vi "Measurement Logic.vi"() -> ()   [LabVIEW 2021, in "audio_frequencyResponseMeasurement.lvlib"]
uses:
  audio_frequencyResponseMeasurement.lvlib
  <vilib>/addons/_NISVFA/_Generation/Signal Generation/SV Discrete Sweep/SV Discrete Sweep.lvclass
  <vilib>/PDM Acquisition Toolkit/host/Classes/Tasks/PCM Input/PCM Input Task.lvclass
  <vilib>/PDM Acquisition Toolkit/host/Classes/Tasks/PCM Input/Controls/DVR PCM Input Task.ctl
  shared/controls/Protocol settings.ctl
  <vilib>/PDM Acquisition Toolkit/host/API/PDM Acquisition Toolkit.lvlib
  <vilib>/PDM Acquisition Toolkit/host/API/Public/Configure/Triggering/Configure PCM Input Trigger (Digital Edge).vi
  <vilib>/PDM Acquisition Toolkit/shared/controls/PXI trigger lines.ctl
  <vilib>/PDM Acquisition Toolkit/shared/PDM Shared.lvlib
  <vilib>/PDM Acquisition Toolkit/shared/controls/trigger polarity.ctl
  <vilib>/PDM Acquisition Toolkit/host/API/Controls/PDM Digital Start Trigger Cluster.ctl
  <resource>/ChannelSupport/_ChannelSupport/_ChannelSupport.lvlib
  <vilib>/DAQmx/configure/events/hardwareSignals.llb/DAQmx Export Signal (Most Signals).vi
  <resource>/objmgr/daqmx.rc
  Program Files/National Instruments/LabVIEW 2021/examples/Sound and Vibration/SoundVib_Audio Examples.lvlib
  <vilib>/DAQmx/write.llb/DAQmx Write (Analog Wfm 1Chan NSamp).vi
  <vilib>/PDM Acquisition Toolkit/host/API/Public/Read/Read PCM Input Waveform.vi
  <vilib>/addons/_NISVFA/_Shared subVIs/Data Objects/Waveforms (DBL)/Waveforms (N Ch).lvclass
  <vilib>/addons/_NISVFA/_Shared subVIs/Data Objects/Waveforms (DBL)/SV Read Next Measurement Data.vi
  C:/Program Files/National Instruments/LabVIEW 2021/vi.lib/addons/_NISVFA/_Generation/Signal Generation/SV Sinusoid/SV Sinusoid.lvclass
  C:/Program Files/National Instruments/LabVIEW 2021/vi.lib/addons/_NISVFA/_Generation/Signal Generation/SV Function/SV Function.lvclass
  C:/Program Files/National Instruments/LabVIEW 2021/vi.lib/addons/_NISVFA/_Generation/Signal Generation/SV Signal/SV Signal.lvclass
  C:/Program Files/National Instruments/LabVIEW 2021/vi.lib/addons/_NISVFA/_Generation/Signal Generation/SV Discrete Sweep/SV Discrete Sweep.lvclass
  Measurement Results.ctl
  <vilib>/PDM Acquisition Toolkit/host/API/Public/Clear/Clear PCM Input Task.vi
  <vilib>/PDM Acquisition Toolkit/host/API/Public/Start/Start PCM Input Task.vi
  Measurement Configuration.ctl
  <vilib>/MeasurementLink/MeasurementLink Measurement Server/Classes/MeasurementContext/MeasurementContext.lvclass
panel:
  out "Measurement Context out":refnum<class "MeasurementContext.lvclass">
  in  "Measurement Context":refnum<class "MeasurementContext.lvclass">
  out "Measurement Results":T1
  in  "Measurement Configuration":T2={"Full scale range"=3.16, "Maximum harmonic"=5, "Analog source resource name"="", "Frequency start"=100.0, "Frequency stop"=20000.0, "Frequency steps"=50, "Frequency spacing"=1, "Amplitude"=1.0, "DC Offset"=0.0, "Measurement duration"=0.001, "Measurement cycles"=10, "Settling time"=0.0, "Settling cycles"=0, "Protocol capture resource name"="", "Data line"=0, "Channel"=0, "Trigger source"=0, "Clock rate"=12288000} {"Settling cycles" min=0 max=5 step=1 format="%.3f"}
  out "error out":errorcluster
  in  "error in":errorcluster
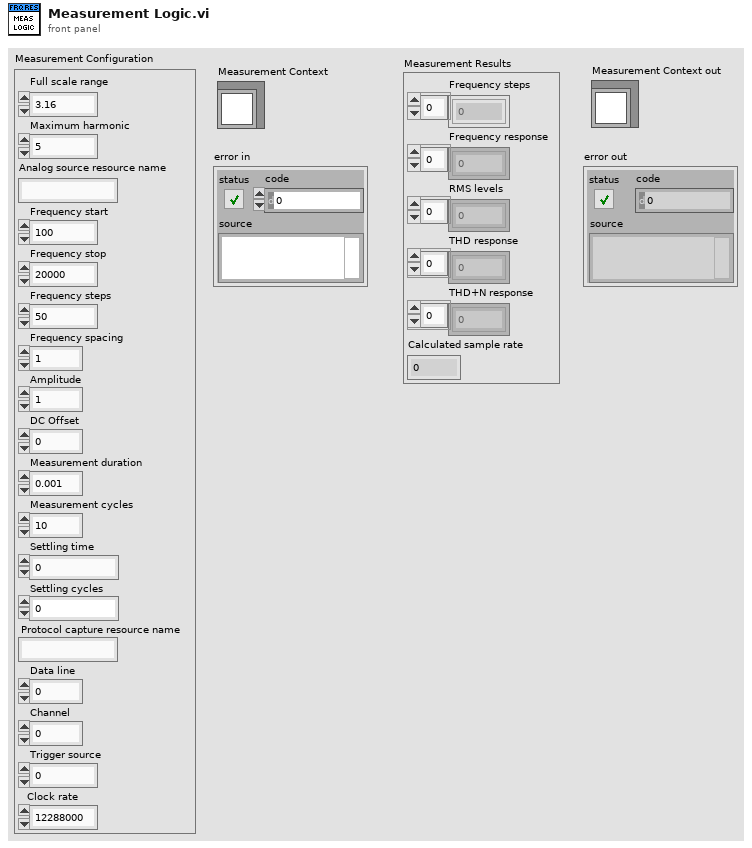
[diagram p1: front panel]
types:
  T1 = typedef "audio_frequencyResponseMeasurement.lvlib/Measurement Results.ctl" = cluster{"Frequency steps":dbl[], "Frequency response":dbl[], "RMS levels":dbl[], "THD response":dbl[], "THD+N response":dbl[], "Calculated sample rate":u32}
  T2 = typedef "audio_frequencyResponseMeasurement.lvlib/Measurement Configuration.ctl" = cluster{"Full scale range":dbl, "Maximum harmonic":i32, "Analog source resource name":string, "Frequency start":dbl, "Frequency stop":dbl, "Frequency steps":i32, "Frequency spacing":u16, "Amplitude":dbl, "DC Offset":dbl, "Measurement duration":dbl, "Measurement cycles":i32, "Settling time":dbl, "Settling cycles":i32, "Protocol capture resource name":string, "Data line":u16, "Channel":u32, "Trigger source":u16, "Clock rate":u32}
  T3 = typedef "PDM Acquisition Class Library.lvlib/PCM Input Task.lvclass/DVR PCM Input Task.ctl" = refnum<data-value>
  T4 = cluster{"signal configuration":refnum<class "SV Discrete Sweep.lvclass">, "ao task":refnum<k21>, "PDM task":T3, "duration":dbl, "samples":i32, "buffer":refnum<data-value>}
  T5 = typedef "PDM Acquisition Toolkit.lvlib/PDM Digital Start Trigger Cluster.ctl" = cluster{"source":T6, "polarity":T7}
  T6 = typedef "PDM Shared.lvlib/PXI trigger lines.ctl" = enum16{"PXI_Trig0", "PXI_Trig1", "PXI_Trig2", "PXI_Trig3", "PXI_Trig4", "PXI_Trig5", "PXI_Trig6", "PXI_Trig7"}
  T7 = typedef "PDM Shared.lvlib/trigger polarity.ctl" = enum16{"Rising Edge", "Falling Edge"}
  T8 = typedef "Protocol settings.ctl" = cluster{"Protocol capture resource name":string, "Data line":u16, "Channel":u32, "Clock rate":u32, "Number of words":i32, "Sensitivity":dbl, "Frame Sync Edge for Channel 0":enum16{"Rising", "Falling"}, "Channel Count Per Frame":u8, "Channel Length":u16, "Bit Depth":u8, "Channel 0 Offset":u16, "Endianness":enum16{"MSB First", "LSB First"}, "Data Justification":enum16{"Left Justified", "Right Justified"}, "Frame Length":u16, "Frame Sync Pulse Width":u16, "Bit Clock Edge  Sync":enum8{"Rising", "Falling"}}
  T9 = cluster{"measured (s)":dbl[], "maximum (samples)":i32}
  T10 = cluster{"RMS level":dbl, "THD":dbl, "THD+N":dbl, "Frequency":dbl}
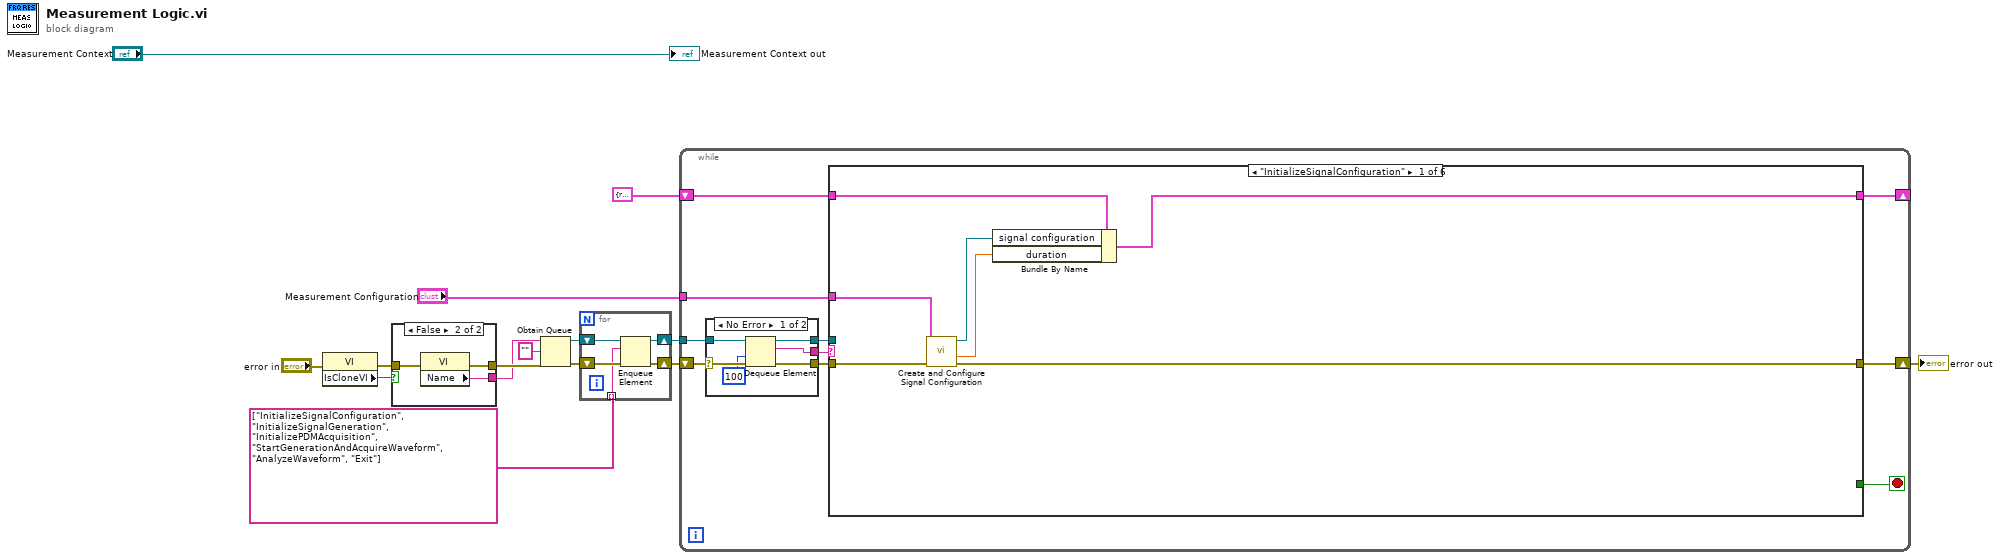
[diagram p0: block diagram]
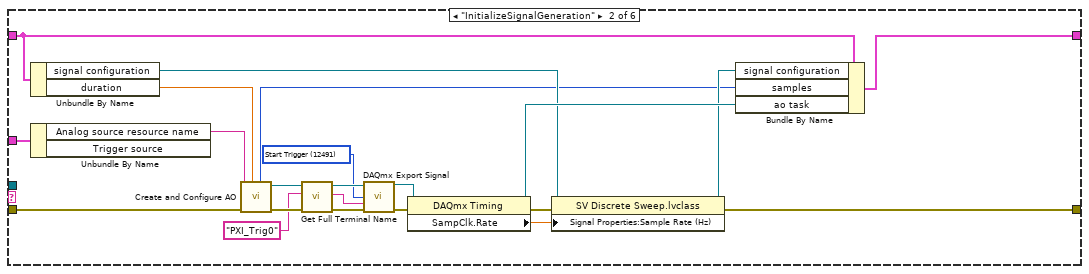
[diagram p2: hidden frame]
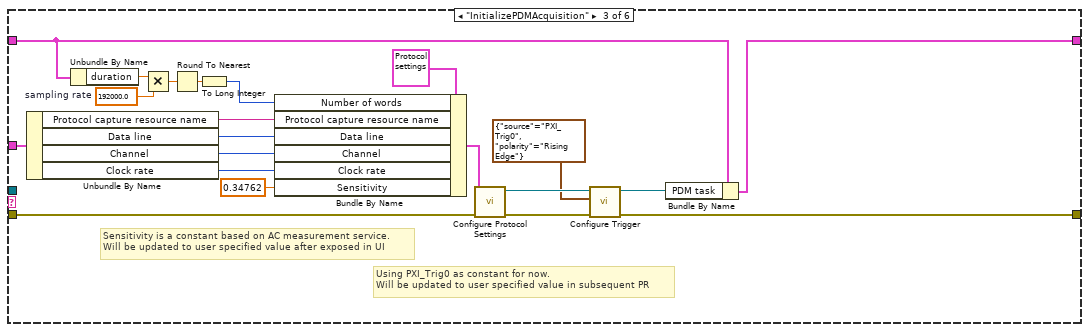
[diagram p3: hidden frame]
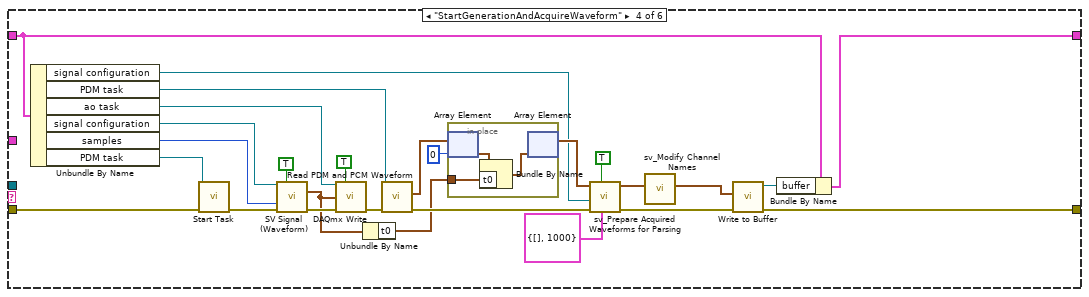
[diagram p4: hidden frame]
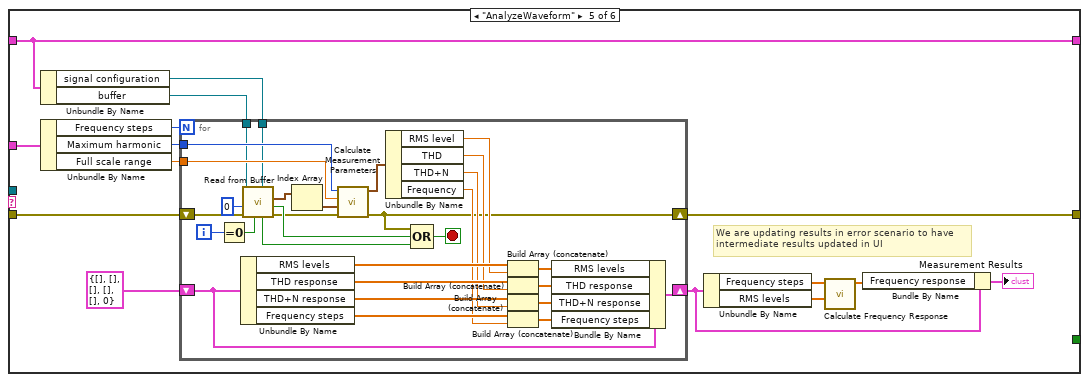
[diagram p5: hidden frame]
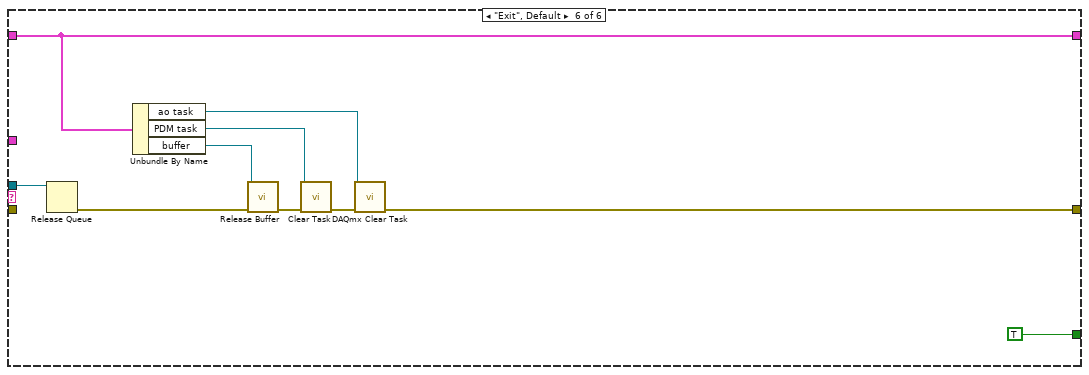
[diagram p6: hidden frame]
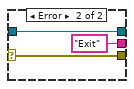
[diagram p7: hidden frame]
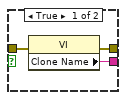
[diagram p8: hidden frame]
diagram:
  n1 = property class="VI"(error in="error in") -> (error out=w11:errorcluster, "IsCloneVI"=w12:bool)  [unwired: 1 in, 1 out]
  n2 = case shown="False" w12 {
    tunnel: [w18 w21] -> w10
    tunnel: [w17 w20] -> w9
    tunnel: w11 -> [w16 w19]
    frame True {
      n3 = property class="VI"(error in=w16) -> (error out=w18:errorcluster, "Clone Name"=w17:string)  [unwired: 1 in, 1 out]
    }
    frame False {
      n4 = property class="VI"(error in=w19) -> (error out=w21:errorcluster, "Name"=w20:string)  [unwired: 1 in, 1 out]
    }
  }
  n5 = Obtain Queue(name (unnamed)=w9, element data type="", error in (no error)=w10) -> (queue out=w13:refnum<queue>, error out=w8:errorcluster)  [unwired: 2 in, 1 out]
  n6 = for {
    shift-right: [w24] -> w5
    shift-left: w13 -> [w26]
    shift-right: [w23] -> w4
    shift-left: w8 -> [w25]
    tunnel: string[] ["InitializeSignalConfiguration", "InitializeSignalGeneration", "InitializePDMAcquisition", "StartGenerationAndAcquireWaveform", "AnalyzeWaveform", "Exit"] ("Step sequence") -> [w22] mode=indexing
    n7 = Enqueue Element(queue=w26, element=w22, error in (no error)=w25) -> (queue out=w24:refnum<queue>, error out=w23:errorcluster)  [unwired: 1 in, 1 out]
  }
  n8 = while {
    tunnel: w5 -> [w36]
    tunnel: "Measurement Configuration" -> [w31]
    shift-right: [w28] -> _
    shift-left: T4 {"signal configuration"=refnum, "ao task"="", "PDM task"=refnum, "duration"=0.0, "samples"=0, "buffer"=refnum} ("output cluster") -> [w29]
    shift-right: [w27] -> w1
    shift-left: w4 -> [w35]
    stop <- w32 stop-if-true
    n9 = case shown="No Error" w35 {
      selector: w35 -> [w175 w179]
      tunnel: w36 -> [w177 w178]
      tunnel: [w176 "Exit" ("t")] -> w34
      tunnel: [w174 w179] -> w30
      tunnel: [w172 w178] -> w33
      frame No Error {
        n10 = Dequeue Element(queue=w177, timeout in ms (-1)=100, error in (no error)=w175) -> (queue out=w172:refnum<queue>, element=w176:string, error out=w174:errorcluster)  [unwired: 1 out]
      }
      frame Error {
      }
    }
    n11 = case shown="\"InitializeSignalConfiguration\"" w34 {
      tunnel: w33 -> [_ _ _ _ _ w171]
      tunnel: [_ _ _ _ _ TRUE] -> w32
      tunnel: w31 -> [w42 w65 w85 _ w130 _]
      tunnel: w30 -> [w43 w63 w86 w88 w131 _]
      tunnel: w29 -> [w41 w62 w74 w91 w125 w169]
      tunnel: [w38 w61 w78 w92 w125 w169] -> w28
      tunnel: [w37 w51 w66 w95 w127 w162] -> w27
      frame "InitializeSignalConfiguration" {
        n12 = call "Create and Configure Signal Configuration.vi"("error in"=w43, "Measurement configuration"=w42) -> ("error out"=w37:errorcluster, "duration"=w39:dbl, "signal configuration"=w40:refnum<class "SV Discrete Sweep.lvclass">)  [unwired: 7 in]
        n13 = Bundle By Name(cluster=w41, "signal configuration"=w40, "duration"=w39) -> (w38:T4)
      }
      frame "InitializeSignalGeneration" {
        w55 = 12491 items=["AI Convert Clock"=12484, "10MHz Reference Clock"=12536, "20MHz Timebase Clock"=12486, "Sample Clock"=12487, "Advance Trigger"=12488, "Reference Trigger"=12490, "Start Trigger"=12491, "Advance Complete Event"=12492, "AI Hold Complete Event"=12493, "Counter Output Event"=12494, "Change Detection Event"=12511, "Watchdog Timer Expired Event"=12512] ("signal")
        n14 = Unbundle By Name(w62) -> ("signal configuration"=w47:refnum<class "SV Discrete Sweep.lvclass">, "duration"=w45:dbl)
        n15 = Unbundle By Name(w65) -> ("Analog source resource name"=w64:string)  [unwired: 1 out]
        n16 = call "Create and Configure AO.vi"("duration"=w45, "error in"=w63, "AO channel"=w64) -> ("error out"=w60:errorcluster, "AO task"=w49:refnum<k21>, "samples"=w44:i32)  [unwired: 6 in]
        n17 = call "Get Full Terminal Name.vi"("error in"=w60, "Local Terminal Name"="PXI_Trig0" ("Trigger line"), "task/channels in"=w49) -> ("error out"=w57:errorcluster, "Terminal Name with Device Prefix"=w56:tag, "task out"=w58:refnum<k21>)  [unwired: 6 in]
        n18 = call-poly <vilib>:"DAQmx Export Signal.vi"("task/channels in"=w58, "signal"=w55, "output terminal"=w56, "error in"=w57) -> ("task out"=w50:refnum<k21>, "error out"=w52:errorcluster)  [unwired: 10 in]
        n19 = property class="DAQmx Timing"(reference=w50, error in=w52) -> (reference out=w48:refnum<k21>, error out=w54:errorcluster, "SampClk.Rate"=w53:dbl)
        n20 = property class="SV Discrete Sweep.lvclass"(reference=w47, error in=w54, "Signal Properties:Sample Rate (Hz)"=w53) -> (reference out=w46:refnum<class "SV Discrete Sweep.lvclass">, error out=w51:errorcluster)
        n21 = Bundle By Name(cluster=w62, "signal configuration"=w46, "samples"=w44, "ao task"=w48) -> (w61:T4)
      }
      frame "InitializePDMAcquisition" {
        w77 = 192000.0  # sampling rate
        # "Using PXI_Trig0 as constant for now.\nWill be updated to user specified value in subsequent PR"
        # "Sensitivity is a constant based on AC measurement service.\nWill be updated to user specified value after exposed in UI"
        n22 = Unbundle By Name(w85) -> ("Protocol capture resource name"=w83:string, "Data line"=w82:u16, "Channel"=w81:u32, "Clock rate"=w80:u32)
        n23 = Unbundle By Name(w74) -> ("duration"=w73:dbl)
        n24 = Multiply(x=w73, y=w77) -> (x*y=w75:dbl)
        n25 = Round To Nearest(number=w75) -> (nearest integer value=w76:dbl)
        n26 = To Long Integer(number=w76) -> (32bit integer=w72:i32)
        n27 = Bundle By Name(cluster=T8 {"Protocol capture resource name"="", "Data line"=0, "Channel"=0, "Clock rate"=12288000, "Number of words"=19200, "Sensitivity"=0.34762, "Frame Sync Edge for Channel 0"=enum."Falling", "Channel Count Per Frame"=2, "Channel Length"=32, "Bit Depth"=24, "Channel 0 Offset"=1, "Endianness"=enum."MSB First", "Data Justification"=enum."Left Justified", "Frame Length"=64, "Frame Sync Pulse Width"=32, "Bit Clock Edge  Sync"=enum."Falling"} ("Protocol settings"), "Number of words"=w72, "Protocol capture resource name"=w83, "Data line"=w82, "Channel"=w81, "Clock rate"=w80, "Sensitivity"=0.34762) -> (w79:T8)
        n28 = call "Configure Protocol Settings.vi"("error in"=w86, "Protocol settings"=w79) -> ("error out"=w69:errorcluster, "PDM task"=w70:T3)  [unwired: 8 in]
        n29 = call-poly <vilib>:"Configure Trigger.vi"("error in"=w69, "trigger configuration"=T5 {"source"=enum."PXI_Trig0", "polarity"=enum."Rising Edge"}, "PCM input task in"=w70) -> ("error out"=w66:errorcluster, "PCM input task out"=w67:T3)  [unwired: 7 in]
        n30 = Bundle By Name(cluster=w74, "PDM task"=w67) -> (w78:T4)
      }
      frame "StartGenerationAndAcquireWaveform" {
        n31 = Unbundle By Name(w91) -> ("signal configuration"=w99:refnum<class "SV Discrete Sweep.lvclass">, "PDM task"=w97:T3, "ao task"=w106:refnum<k21>, "signal configuration"=w98:refnum<class "SV Discrete Sweep.lvclass">, "samples"=w100:i32, "PDM task"=w87:T3)
        n32 = call-poly <vilib>:"Start Task.vi"("error in"=w88, "PCM input task in"=w87) -> ("error out"=w89:errorcluster)  [unwired: 8 in, 1 out]
        n33 = call-dynamic "SV Signal (Waveform).vi"("signal configuration"=w98, "reset"=TRUE, "samples"=w100, "error in (no error)"=w89) -> ("output waveform"=w109:waveform(dbl), "error out"=w112:errorcluster)  [unwired: 6 in, 4 out]
        n34 = call-poly <vilib>:"DAQmx Write.vi"("task/channels in"=w106, "auto start"=TRUE, "data"=w109, "error in"=w112) -> ("error out"=w110:errorcluster)  [unwired: 9 in, 2 out]
        n35 = Unbundle By Name(w109) -> ("t0"=w103:timestamp)
        n36 = call-poly <vilib>:"Read PDM and PCM Waveform.vi"("error in"=w110, "PCM input task In"=w97) -> ("error out"=w108:errorcluster, "PCM waveforms"=w105:waveform(dbl)[])  [unwired: 4 in, 4 out]
        n37 = in-place {
          in-place-border: w103 -> [w115]
          n38 = in-place-array #1(w105, 0) -> (w116:waveform(dbl))
          n39 = Bundle By Name(cluster=w116, "t0"=w115) -> (w114:waveform(dbl))
          n40 = in-place-array #1(w114) -> (w102:waveform(dbl)[])  [unwired: 1 out]
        }
        n41 = call "sv_Prepare Acquired Waveforms for Parsing.vi"("propagation delay"=T9 {"measured (s)"=[], "maximum (samples)"=1000}, "restart (F)"=TRUE, "error in"=w108, "SV Signal"=w99, "acquired channel waveforms"=w102) -> ("error out"=w96:errorcluster, "aligned channel waveforms"=w101:waveform(dbl)[])  [unwired: 4 in, 1 out]
        n42 = call "sv_Modify Channel Names.vi"("waveforms"=w101) -> ("renamed waveforms"=w94:waveform(dbl)[])  [unwired: 8 in]
        n43 = call <vilib>:"Write to Buffer.vi"("error in (no error)"=w96, "waveforms"=w94) -> ("error out"=w95:errorcluster, "buffer out"=w93:refnum<data-value>)  [unwired: 7 in, 1 out]
        n44 = Bundle By Name(cluster=w91, "buffer"=w93) -> (w92:T4)
      }
      frame "AnalyzeWaveform" {
        # "We are updating results in error scenario to have\nintermediate results updated in UI"
        n45 = Unbundle By Name(w125) -> ("signal configuration"=w123:refnum<class "SV Discrete Sweep.lvclass">, "buffer"=w124:refnum<data-value>)
        n46 = Unbundle By Name(w130) -> ("Frequency steps"=w126:i32, "Maximum harmonic"=w128:i32, "Full scale range"=w129:dbl)
        n47 = for {
          N: w126 -> [_]
          tunnel: w129 -> [w161]
          tunnel: w128 -> [w160]
          shift-right: [w133] -> w127
          shift-left: w131 -> [w159]
          tunnel: w124 -> [w156]
          tunnel: w123 -> [w154]
          shift-right: [w137] -> w119
          shift-left: T1 {"Frequency steps"=[], "Frequency response"=[], "RMS levels"=[], "THD response"=[], "THD+N response"=[], "Calculated sample rate"=0} ("Measurement Results") -> [w142]
          i -> [w158]
          stop <- w132 stop-if-true
          n48 = Equal To 0?(x=w158) -> (x = 0?=w157:bool)
          n49 = Unbundle By Name(w142) -> ("RMS levels"=w150:dbl[], "THD response"=w148:dbl[], "THD+N response"=w146:dbl[], "Frequency steps"=w144:dbl[])
          n50 = call-poly <vilib>:"Read from Buffer.vi"("test signal configuration"=w154, "reset start (F)"=w157, "error in (no error)"=w159, "timeout (1000 ms)"=0, "buffer"=w156) -> ("error out"=w134:errorcluster, "end of buffer"=w136:bool, "waveforms subset"=w153:waveform(dbl)[], "done"=w135:bool)  [unwired: 2 in, 1 out]
          n51 = Index Array(array=w153) -> (element=w152:waveform(dbl))  [unwired: 1 in]
          n52 = call "Calculate Measurement Parameters.vi"("error in"=w134, "scaled signal in [EU]"=w152, "Full scale range"=w161, "Maximum harmonic"=w160) -> ("error out"=w133:errorcluster, "Meas results"=w151:T10)  [unwired: 6 in]
          n53 = Unbundle By Name(w151) -> ("RMS level"=w149:dbl, "THD"=w147:dbl, "THD+N"=w145:dbl, "Frequency"=w143:dbl)
          n54 = Compound Arithmetic op=OR(w133, w136, w135) -> (w132:bool)
          n55 = Build Array (concatenate)(w150, w149) -> (w141:dbl[])
          n56 = Build Array (concatenate)(w148, w147) -> (w140:dbl[])
          n57 = Build Array (concatenate)(w146, w145) -> (w139:dbl[])
          n58 = Build Array (concatenate)(w144, w143) -> (w138:dbl[])
          n59 = Bundle By Name(cluster=w142, "RMS levels"=w141, "THD response"=w140, "THD+N response"=w139, "Frequency steps"=w138) -> (w137:T1)
        }
        n60 = Unbundle By Name(w119) -> ("Frequency steps"=w121:dbl[], "RMS levels"=w120:dbl[])
        n61 = call "Calculate Frequency Response.vi"("Amplitudes"=w120, "Frequencies"=w121) -> ("Frequency response @ 1KHz"=w118:dbl[])  [unwired: 9 in]
        n62 = Bundle By Name(cluster=w119, "Frequency response"=w118) -> (→"Measurement Results":T1)
      }
      frame "Exit", Default {
        n63 = Release Queue(queue=w171) -> (error out=w167:errorcluster)  [unwired: 2 in, 2 out]
        n64 = Unbundle By Name(w169) -> ("ao task"=w163:refnum<k21>, "PDM task"=w165:T3, "buffer"=w168:refnum<data-value>)
        n65 = call <vilib>:"Release Buffer.vi"("error in (no error)"=w167, "buffer"=w168) -> ("error out"=w166:errorcluster)  [unwired: 9 in]
        n66 = call-poly <vilib>:"Clear Task.vi"("error in"=w166, "PCM input task in"=w165) -> ("error out"=w164:errorcluster)  [unwired: 9 in]
        n67 = call <vilib>:"DAQmx Clear Task.vi"("task in"=w163, "error in"=w164) -> ("error out"=w162:errorcluster)  [unwired: 13 in]
      }
    }
  }
  "error out" <- w1
  "Measurement Context out" <- "Measurement Context"
